vi "EXPRES Parse Message.vi"(8 "error in (no error)":errorcluster, 9 "queue":refnum<queue>, 10 "JSON string":string, 11 "method":string) -> (0 "error out":errorcluster)   [LabVIEW 2016]
uses:
  Controls/Message Structure.ctl
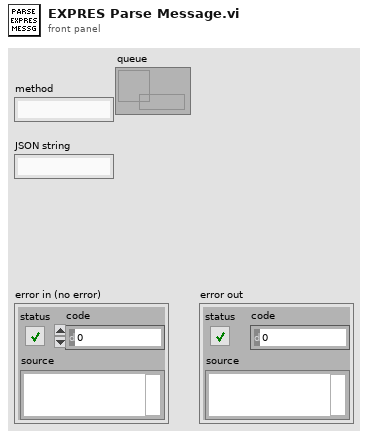
[diagram p1: front panel]
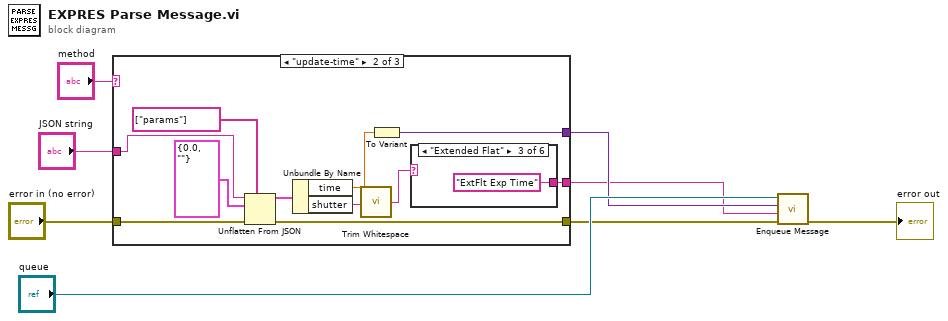
[diagram p0: block diagram]
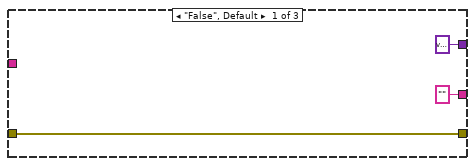
[diagram p2: hidden frame]
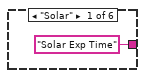
[diagram p3: hidden frame]
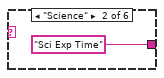
[diagram p4: hidden frame]
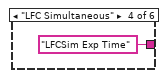
[diagram p5: hidden frame]
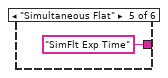
[diagram p6: hidden frame]
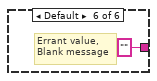
[diagram p7: hidden frame]
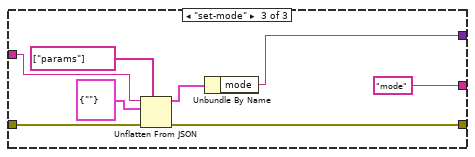
[diagram p8: hidden frame]
diagram:
  n1 = case shown="\"update-time\"" "method" {
    tunnel: [w11 w21 w34] -> w2
    tunnel: "error in (no error)" -> [w11 w22 w35]
    tunnel: "JSON string" -> [_ w18 w33]
    tunnel: [variant ("Variant") w16 w30] -> w4
    tunnel: ["" w12 "mode"] -> w3
    frame "False", Default {
    }
    frame "update-time" {
      n2 = Unflatten From JSON(path=string[] ["params"], JSON string=w18, type and defaults=cluster{"time":dbl, "shutter":string} {"time"=0.0, "shutter"=""} ("params"), error in (no error)=w22) -> (value=w17:cluster{"time":dbl, "shutter":string}, error out=w21:errorcluster)  [unwired: 3 in]
      n3 = Unbundle By Name(w17) -> ("time"=w15:dbl, "shutter"=w14:string)
      n4 = call <vilib>:"Trim Whitespace.vi"("string"=w14) -> ("trimmed string"=w13:string)  [unwired: 1 in]
      n5 = To Variant(anything=w15) -> (Variant=w16:variant)
      n6 = case shown="\"Extended Flat\"" w13 {
        tunnel: ["Solar Exp Time" "Sci Exp Time" "ExtFlt Exp Time" "LFCSim Exp Time" "SimFlt Exp Time" ""] -> w12
        frame "Solar" {
        }
        frame "Science" {
        }
        frame "Extended Flat" {
        }
        frame "LFC Simultaneous" {
        }
        frame "Simultaneous Flat" {
        }
        frame Default {
          # "Errant value, \nBlank message"
        }
      }
    }
    frame "set-mode" {
      n7 = Unflatten From JSON(path=string[] ["params"], JSON string=w33, type and defaults=cluster{"mode":string} {"mode"=""} ("params"), error in (no error)=w35) -> (value=w31:cluster{"mode":string}, error out=w34:errorcluster)  [unwired: 3 in]
      n8 = Unbundle By Name(w31) -> ("mode"=w30:string)
    }
  }
  n9 = call "Enqueue Message.vi"("error in (no error)"=w2, "Cmd"=w3, "Data variant"=w4, "Queue In"="queue") -> ("error out"=→"error out":errorcluster)  [unwired: 7 in]
